vi "IMUprocess.vi"(9 "Frames Read":u16[](array[numeric]), 11 "error in (no error)":errorcluster) -> (0 "error out":errorcluster, 2 "Gyro deg/s":dbl[](array[numeric]), 3 "Accel g's":dbl[](array[numeric]))   [LabVIEW 2016]
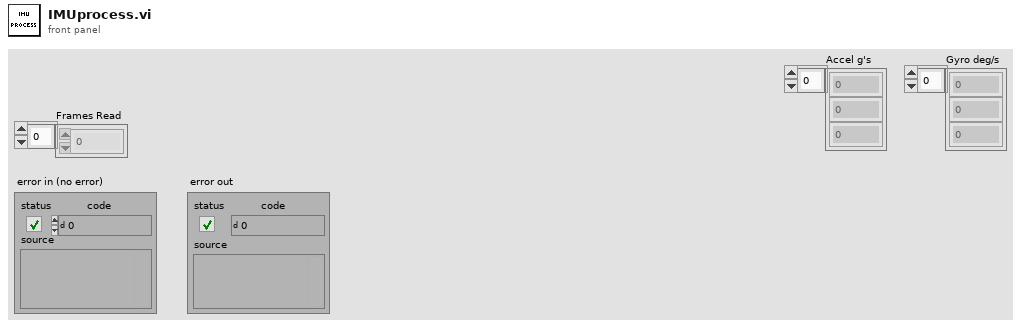
[diagram p1: front panel]
types:
  T1 = cluster{"X gyro bias":dbl, "Y gyro bias":dbl, "Z gyro bias":dbl, "X acc bias":dbl, "Y acc bias":dbl, "Z acc bias":dbl}
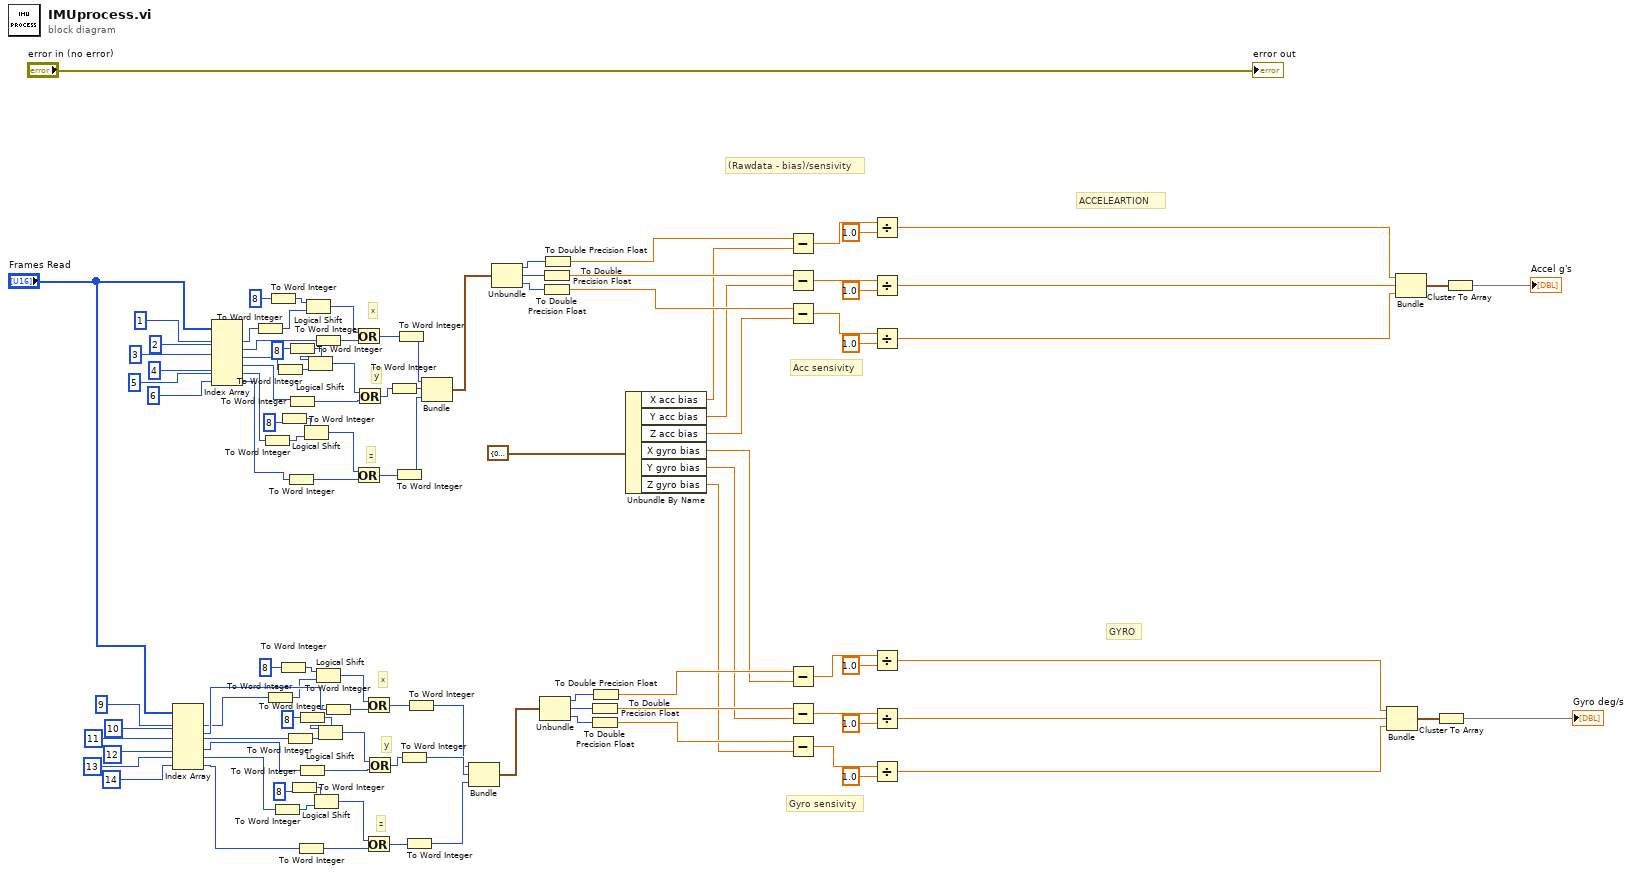
[diagram p0: block diagram]
diagram:
  # "Gyro sensivity"
  # "(Rawdata - bias)/sensivity"
  # "GYRO"
  # "ACCELEARTION"
  # "Acc sensivity"
  # "z"
  # "y"
  # "x"
  # "z"
  # "y"
  # "x"
  n1 = Index Array(array="Frames Read", index #1=9 ("index"), index #2=10 ("index"), index #3=11 ("index"), index #4=12 ("index"), index #5=13 ("index"), index #6=14 ("index")) -> (element #1=w95:u16, element #2=w96:u16, element #3=w97:u16, element #4=w98:u16, element #5=w99:u16, element #6=w100:u16)
  n2 = Index Array(array="Frames Read", index #1=1 ("index"), index #2=2 ("index"), index #3=3 ("index"), index #4=4 ("index"), index #5=5 ("index"), index #6=6 ("index")) -> (element #1=w52:u16, element #2=w57:u16, element #3=w65:u16, element #4=w69:u16, element #5=w74:u16, element #6=w75:u16)
  n3 = To Word Integer(number=w52) -> (16bit integer=w53:i16)
  n4 = To Word Integer(number=w74) -> (16bit integer=w73:i16)
  n5 = To Word Integer(number=w95) -> (16bit integer=w88:i16)
  n6 = To Word Integer(number=i16 8 ("y")) -> (16bit integer=w54:i16)
  n7 = To Word Integer(number=w99) -> (16bit integer=w78:i16)
  n8 = To Word Integer(number=w65) -> (16bit integer=w68:i16)
  n9 = To Word Integer(number=i16 8 ("y")) -> (16bit integer=w87:i16)
  n10 = To Word Integer(number=i16 8 ("y")) -> (16bit integer=w72:i16)
  n11 = To Word Integer(number=w97) -> (16bit integer=w82:i16)
  n12 = To Word Integer(number=w75) -> (16bit integer=w76:i16)
  n13 = To Word Integer(number=i16 8 ("y")) -> (16bit integer=w67:i16)
  n14 = To Word Integer(number=w69) -> (16bit integer=w70:i16)
  n15 = To Word Integer(number=i16 8 ("y")) -> (16bit integer=w79:i16)
  n16 = To Word Integer(number=w100) -> (16bit integer=w77:i16)
  n17 = To Word Integer(number=i16 8 ("y")) -> (16bit integer=w83:i16)
  n18 = To Word Integer(number=w98) -> (16bit integer=w81:i16)
  n19 = Logical Shift(y=w72, x=w73) -> (x << y=w37:i16)
  n20 = Logical Shift(y=w54, x=w53) -> (x << y=w35:i16)
  n21 = Logical Shift(y=w67, x=w68) -> (x << y=w36:i16)
  n22 = Logical Shift(y=w79, x=w78) -> (x << y=w92:i16)
  n23 = To Word Integer(number=w57) -> (16bit integer=w56:i16)
  n24 = Logical Shift(y=w87, x=w88) -> (x << y=w94:i16)
  n25 = Logical Shift(y=w83, x=w82) -> (x << y=w93:i16)
  n26 = To Word Integer(number=w96) -> (16bit integer=w85:i16)
  n27 = Or(x=w35, y=w56) -> (x .or. y?=w46:i16)
  n28 = Or(x=w37, y=w76) -> (x .or. y?=w49:i16)
  n29 = Or(x=w36, y=w70) -> (x .or. y?=w50:i16)
  n30 = Or(x=w94, y=w85) -> (x .or. y?=w91:i16)
  n31 = Or(x=w92, y=w77) -> (x .or. y?=w90:i16)
  n32 = Or(x=w93, y=w81) -> (x .or. y?=w89:i16)
  n33 = To Word Integer(number=w50) -> (16bit integer=w48:i16)
  n34 = To Word Integer(number=w49) -> (16bit integer=w51:i16)
  n35 = To Word Integer(number=w46) -> (16bit integer=w47:i16)
  n36 = To Word Integer(number=w89) -> (16bit integer=w102:i16)
  n37 = To Word Integer(number=w90) -> (16bit integer=w103:i16)
  n38 = To Word Integer(number=w91) -> (16bit integer=w101:i16)
  n39 = Bundle(w47, w48, w51) -> (w45:cluster{i16, i16, i16})  [unwired: 1 in]
  n40 = Bundle(w101, w102, w103) -> (w64:cluster{i16, i16, i16})  [unwired: 1 in]
  n41 = Unbundle(w45) -> (w58:i16, w59:i16, w60:i16)
  n42 = Unbundle(w64) -> (w63:i16, w62:i16, w61:i16)
  n43 = To Double Precision Float(number=w59) -> (double precision float=w109:dbl)
  n44 = To Double Precision Float(number=w60) -> (double precision float=w110:dbl)
  n45 = To Double Precision Float(number=w58) -> (double precision float=w27:dbl)
  n46 = To Double Precision Float(number=w62) -> (double precision float=w4:dbl)
  n47 = To Double Precision Float(number=w61) -> (double precision float=w5:dbl)
  n48 = To Double Precision Float(number=w63) -> (double precision float=w6:dbl)
  n49 = Unbundle By Name(T1 {"X gyro bias"=0.0, "Y gyro bias"=0.0, "Z gyro bias"=0.0, "X acc bias"=0.0, "Y acc bias"=0.0, "Z acc bias"=0.0} ("input cluster")) -> ("X acc bias"=w20:dbl, "Y acc bias"=w19:dbl, "Z acc bias"=w18:dbl, "X gyro bias"=w3:dbl, "Y gyro bias"=w2:dbl, "Z gyro bias"=w1:dbl)
  n50 = Subtract(x=w27, y=w20) -> (x-y=w26:dbl)
  n51 = Subtract(x=w109, y=w19) -> (x-y=w25:dbl)
  n52 = Subtract(x=w110, y=w18) -> (x-y=w22:dbl)
  n53 = Subtract(x=w6, y=w3) -> (x-y=w13:dbl)
  n54 = Subtract(x=w4, y=w2) -> (x-y=w12:dbl)
  n55 = Subtract(x=w5, y=w1) -> (x-y=w8:dbl)
  n56 = Divide(x=w26, y=1.0 ("Acc s")) -> (x/y=w104:dbl)
  n57 = Divide(x=w25, y=1.0) -> (x/y=w105:dbl)
  n58 = Divide(x=w22, y=1.0) -> (x/y=w106:dbl)
  n59 = Divide(x=w13, y=1.0 ("Acc s")) -> (x/y=w14:dbl)
  n60 = Divide(x=w12, y=1.0) -> (x/y=w15:dbl)
  n61 = Divide(x=w8, y=1.0) -> (x/y=w16:dbl)
  n62 = Bundle(w14, w15, w16) -> (w17:cluster{dbl, dbl, dbl})  [unwired: 1 in]
  n63 = Bundle(w104, w105, w106) -> (w108:cluster{dbl, dbl, dbl})  [unwired: 1 in]
  n64 = Cluster To Array(cluster=w17) -> (array=→"Gyro deg/s":dbl[])
  n65 = Cluster To Array(cluster=w108) -> (array=→"Accel g's":dbl[])
  "error out" <- "error in (no error)"
